vi "APC_ClearErrorButton.vi"() -> ()   [LabVIEW 2020]
panel:
  in  "Cancel Button":bool
  in  "OK Button":bool
  # "You are about to clear all errors and warnings. Please confirm the operation"
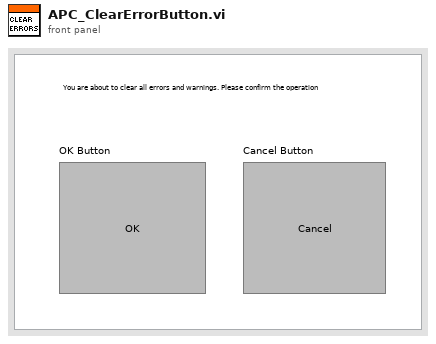
[diagram p1: front panel]
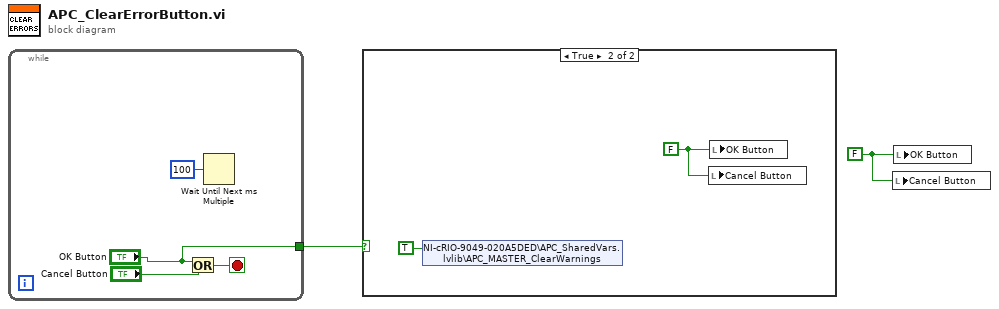
[diagram p0: block diagram]
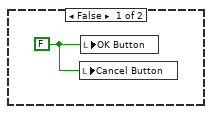
[diagram p2: hidden frame]
diagram:
  w1 = FALSE ("OK Button")
  n1 = while {
    tunnel: ["OK Button"] -> w2
    stop <- w6 stop-if-true
    n2 = Or(x="OK Button", y="Cancel Button") -> (x .or. y?=w6:bool)
    n3 = Wait Until Next ms Multiple(millisecond multiple=u32 100) -> ()  [unwired: 1 out]
  }
  n4 = case shown="True" w2 {
    frame False {
      w7 = FALSE ("OK Button")
      n5 = local write "Cancel Button"(w7) -> ()
      n6 = local write "OK Button"(w7) -> ()
    }
    frame True {
      w9 = FALSE ("OK Button")
      n7 = shared-variable "NI-cRIO-9049-020A5DED\\APC_SharedVars.lvlib\\APC_MASTER_ClearWarnings"(TRUE ("Clear9056warnings")) -> ()  [unwired: 1 in, 1 out]
      n8 = local write "Cancel Button"(w9) -> ()
      n9 = local write "OK Button"(w9) -> ()
    }
  }
  n10 = local write "Cancel Button"(w1) -> ()
  n11 = local write "OK Button"(w1) -> ()
